vi "RT_Coriolis_Force_in_DLR_Navigation_Reference_System_2(SubVI).vi"(0 "Data":dbl[][](array[numeric]), 5 "i":i32, 7 "Vehicle Parameters":T2, 11 "Rotation":T1) -> (4 "Fco (N)":dbl[](array[numeric]))   [LabVIEW 2017]
uses:
  <vilib>/Analysis/baseanly.llb/Real A x B.vi
  <vilib>/Analysis/Matrix/Numeric/Conversions/Array To Matrix - RA.vi
  <vilib>/Analysis/Matrix/Numeric/Conversions/Array To Matrix - RA2.vi
  <vilib>/Analysis/Matrix/Numeric/Conversions/Matrix To Array - RM.vi
  <vilib>/Analysis/NI_AALBase.lvlib
  <vilib>/Analysis/Matrix/NI_Matrix.lvlib
  <vilib>/Analysis/NI_AALPro.lvlib
panel:
  out "OMEGA":dbl[](array[numeric])
  out "m":dbl
  out "Re":dbl[](array[numeric])
  out "re":dbl
  out "CoG (m)":dbl
  out "M_p (kg/s)":dbl
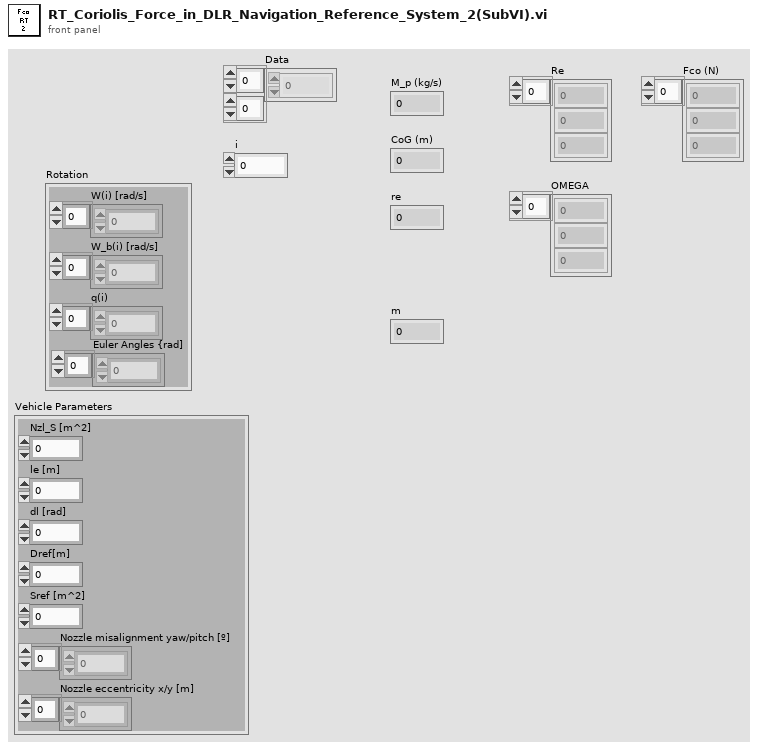
[diagram p1: front panel]
types:
  T1 = cluster{"W(i) [rad/s]":dbl[], "W_b(i) [rad/s]":dbl[], "q(i)":dbl[], "Euler Angles {rad]":dbl[]}
  T2 = cluster{"Nzl_S [m^2]":dbl, "le [m]":dbl, "dl [rad]":dbl, "Dref[m]":dbl, "Sref [m^2]":dbl, "Nozzle misalignment yaw/pitch [º]":dbl[], "Nozzle eccentricity x/y [m]":dbl[]}
  T3 = typedef "NI_Matrix.lvlib/RealMatrix.ctl" = dbl[][]
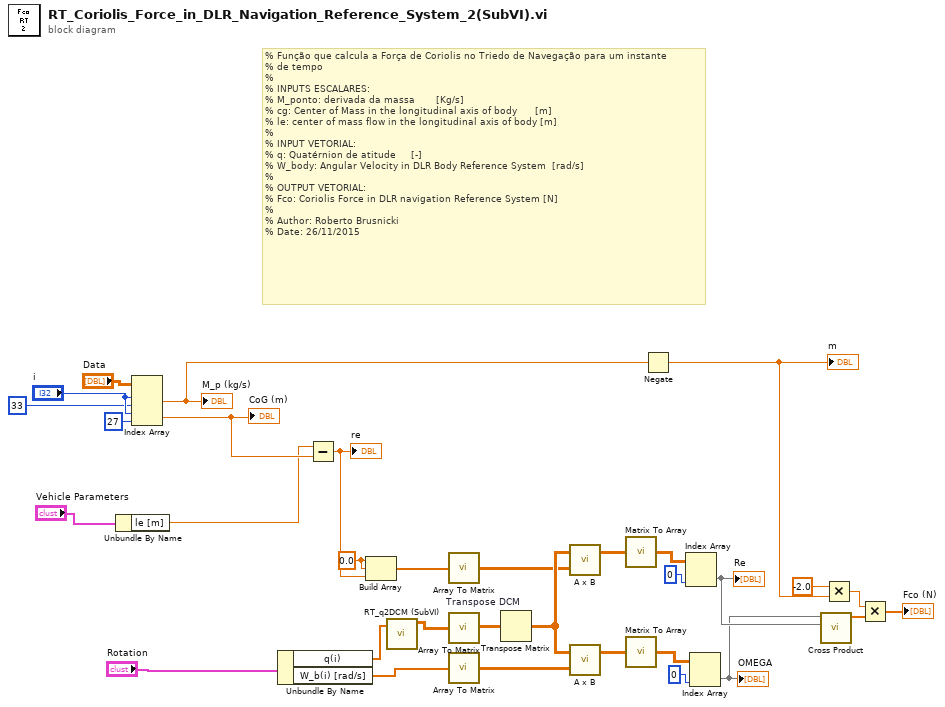
[diagram p0: block diagram]
diagram:
  w18 = 0.0 ("element")
  # "% Função que calcula a Força de Coriolis no Triedo de Navegação para um instante\n% de tempo\n%\n% INPUTS ESCALARES:\n% M_ponto: derivada da massa\t\t\t\t   [Kg/s]\n% cg: Center of Mass in the longitudinal axis of body      [m]\n% le: center of mass flow in the longitudinal axis of body [m]\n% \n% INPUT VETORIAL:\n% q: Quatérnion de atitude\t\t\t\t [-]\n% W_body: Angular Velocity in DLR Body Reference System  [rad/s] \t\n%\n% OUTPUT VETORIAL:\n% Fco: Coriolis Force in DLR navigation Reference System [N]\n%\n% Author: Roberto Brusnicki\n% Date: 26/11/2015"
  n1 = Unbundle By Name("Vehicle Parameters") -> ("le [m]"=w5:dbl)
  n2 = Index Array(array="Data", index (row) #1="i", index (col) #1=33 ("disabled index (col)"), index (row) #2="i", index (col) #2=27 ("disabled index (col)")) -> (element #1=w21:dbl, element #2=w13:dbl)
  "M_p (kg/s)" <- w21
  "CoG (m)" <- w13
  n3 = Unbundle By Name("Rotation") -> ("q(i)"=w3:dbl[], "W_b(i) [rad/s]"=w6:dbl[])
  n4 = Subtract(x=w5, y=w13) -> (x-y=w17:dbl)
  "re" <- w17
  n5 = Build Array(w18, w18, w17) -> (w19:dbl[])
  n6 = call "RT_q2DCM (SubVI).vi"("Quaternion"=w3) -> ("DCM"=w2:dbl[][])  [unwired: 10 in]
  n7 = call-poly <vilib>:"Array To Matrix.vi"("Real 1D Array"=w19) -> ("Real Matrix (Column Vector)"=w16:T3)
  n8 = call-poly <vilib>:"Array To Matrix.vi"("Real 2D Array"=w2) -> ("Real Matrix"=w20:T3)
  n9 = call-poly <vilib>:"Array To Matrix.vi"("Real 1D Array"=w6) -> ("Real Matrix (Column Vector)"=w22:T3)
  n10 = Transpose Matrix "Transpose DCM"(1:w20) -> (0:w25:T3)
  n11 = call-poly <vilib>:"A x B.vi"("B"=w16, "A"=w25) -> ("A x B"=w14:T3)  [unwired: 1 out]
  n12 = call-poly <vilib>:"A x B.vi"("B"=w22, "A"=w25) -> ("A x B"=w24:T3)  [unwired: 1 out]
  n13 = call-poly <vilib>:"Matrix To Array.vi"("Real Matrix"=w14) -> ("Real 2D Array"=w15:dbl[][])
  n14 = call-poly <vilib>:"Matrix To Array.vi"("Real Matrix"=w24) -> ("Real 2D Array"=w23:dbl[][])
  n15 = Negate(x=w21) -> (-x=w28:dbl)
  "m" <- w28
  n16 = Index Array(array=w15, index (col)=0 ("index (row)")) -> (element=w27:dbl[])  [unwired: 1 in]
  "Re" <- w27
  n17 = Index Array(array=w23, index (col)=0 ("index (row)")) -> (element=w26:dbl[])  [unwired: 1 in]
  "OMEGA" <- w26
  n18 = call <vilib>:"Cross Product.vi"("B Vector"=w27, "A Vector"=w26) -> ("Cross Product"=w31:dbl[])  [unwired: 8 in, 1 out]
  n19 = Multiply(x=-2.0, y=w28) -> (x*y=w30:dbl)
  n20 = Multiply(x=w30, y=w31) -> (x*y=→"Fco (N)":dbl[])
